vi "ShooterButton.vi"(10 "Action":T1, 11 "Input":bool) -> ()   [LabVIEW 2013]
doc: "Send comand to the shooter subsystem when the rising edge of a button is detected."
uses:
  ShooterCmds.ctl
  ShooterStates.ctl
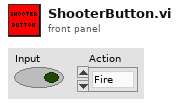
[diagram p1: front panel]
types:
  T1 = typedef "ShooterCmds.ctl" = enum16{"Fire", "Lob", "Retract", "End Of Match", "Release", "FireAuto"}
  T2 = typedef "ShooterStates.ctl" = enum16{"Init", "Ready", "RetractFull", "Disengage Clutch", "Clutch Delay", "Fire", "Fire Delay", "Latch", "Retract", "Release"}
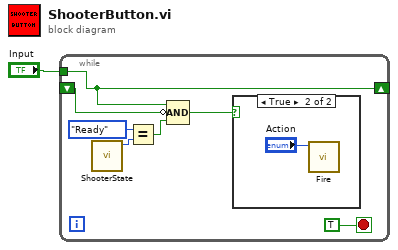
[diagram p0: block diagram]
diagram:
  n1 = while {
    shift-right: [w7] -> _
    shift-left: _ -> [w4]
    tunnel: "Input" -> [w7]
    stop <- TRUE stop-if-true
    n2 = call "ShooterState.vi"() -> ("Value out"=w5:T2)  [unwired: 11 in]
    n3 = Equal?(x=ShooterStates."Ready", y=w5) -> (x = y?=w2:bool)
    n4 = Compound Arithmetic op=AND(w7, invert w4, w2) -> (w6:bool)
    n5 = case shown="True" w6 {
      frame False {
      }
      frame True {
        n6 = call "Fire.vi"(11:"Action") -> ()  [unwired: 10 in, 1 out]
      }
    }
  }
